vi "Classify Error.vi"(10 "Error Code":i32) -> (2 "Error Classification":i32)   [LabVIEW 2018, in "Counter.lvlib" / "PICOTEST U62XXA series.lvlib"]
doc: "This VI is used to check error code."
uses:
  PICOTEST U62XXA series.lvlib
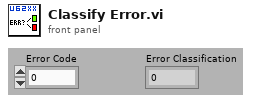
[diagram p1: front panel]
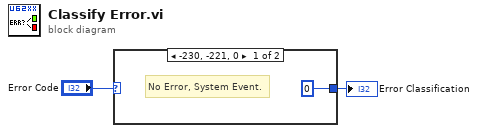
[diagram p0: block diagram]
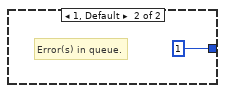
[diagram p2: hidden frame]
diagram:
  n1 = case shown="-230, -221, 0" "Error Code" {
    tunnel: [0 1] -> w1
    frame -230, -221, 0 {
      # "No Error, System Event."
    }
    frame 1, Default {
      # "Error(s) in queue."
    }
  }
  "Error Classification" <- w1
